vi "Speed.vi"(3 "Speed1":dbl, 7 "LabVIEW Web Service Request":refnum<class "Web Request.lvclass">) -> ()   [LabVIEW 2014]
uses:
  <vilib>/wsapi/Web Request.lvclass
  controls/UI DataSam.ctl
panel:
  # "Use the Web Service Request input terminal to call the VIs on the Web Services palette. Do not remove it from the connector pane unless you don't need access to the palette."
  # "Each additional control wired to the connector pane will be available as an input in the URL. To include an indicator in terminal-mode output (the default setting), it must also be wired to the connector pane."
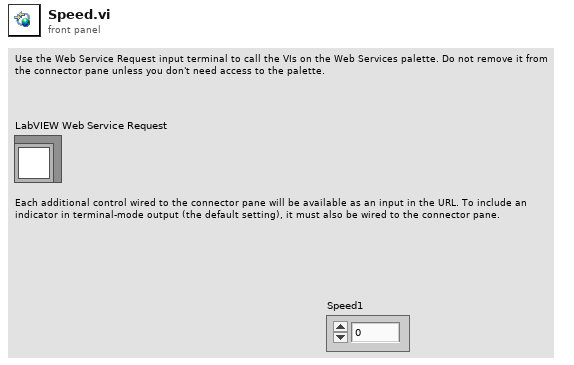
[diagram p1: front panel]
types:
  T1 = typedef "UI DataSam.ctl" = cluster{"Message":string, "Data":variant}
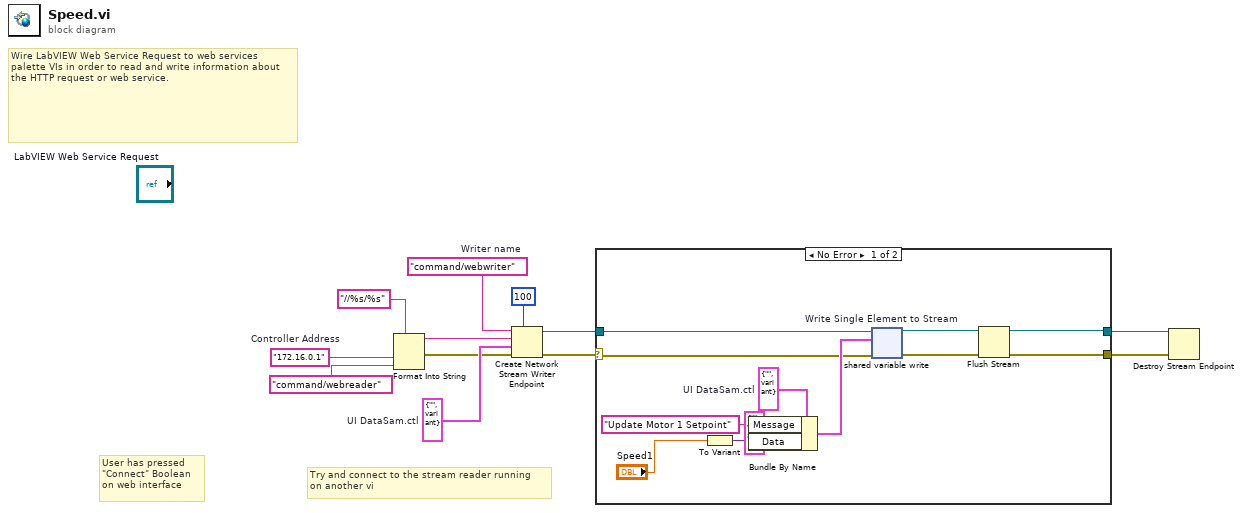
[diagram p0: block diagram]
diagram:
  w12 = "172.16.0.1"  # Controller Address
  w9 = T1 {"Message"="", "Data"=variant}  # UI DataSam.ctl
  w8 = "command/webwriter"  # Writer name
  (unwired) T1 {"Message"="", "Data"=variant} ("UI DataSam.ctl")
  # "Try and connect to the stream reader running\non another vi"
  # "User has pressed\n\"Connect\" Boolean\non web interface"
  # "Wire LabVIEW Web Service Request to web services palette VIs in order to read and write information about the HTTP request or web service."
  n1 = Format Into String(format string="//%s/%s", w12, "command/webreader" ("input 2")) -> (resulting string=w6:string, error out=w5:errorcluster)  [unwired: 2 in]
  n2 = Create Network Stream Writer Endpoint(7:100 ("writer buffer size"), 8:w5, 9:w9, 10:w6, 11:w8) -> (0:w11:errorcluster, 3:w10:refnum<k21>)  [unwired: 2 in]
  n3 = case shown="No Error" w11 {
    selector: w11 -> [w14 w24]
    tunnel: w10 -> [w19 w25]
    tunnel: [w18 w25] -> w2
    tunnel: [w17 w24] -> w1
    frame No Error {
      w16 = T1 {"Message"="", "Data"=variant}  # UI DataSam.ctl
      n4 = To Variant(anything="Speed1") -> (Variant=w23:variant)
      n5 = Bundle By Name(cluster=w16, "Message"="Update Motor 1 Setpoint", "Data"=w23) -> (w15:T1)
      n6 = shared-variable-write "Write Single Element to Stream"(w19, w14, w15) -> (w21:refnum<k21>, w20:errorcluster)  [unwired: 1 in, 1 out]
      n7 = Flush Stream(8:w20, 11:w21) -> (0:w17:errorcluster, 3:w18:refnum<k21>)  [unwired: 2 in, 1 out]
    }
    frame Error {
    }
  }
  n8 = Destroy Stream Endpoint(8:w1, 11:w2) -> ()  [unwired: 1 out]
